vi "BUILD_install and upload core.vi"(7 "buildlog":path, 9 "LabVIEW Version":string, 10 "Repository Name":string, 11 "appended path":path) -> (0 "error out":errorcluster)   [LabVIEW 2013]
uses:
  <vilib>/JKI/VIPM API/VIPM API_vipm_api.lvlib
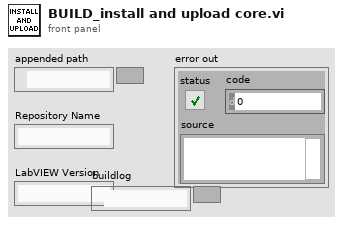
[diagram p1: front panel]
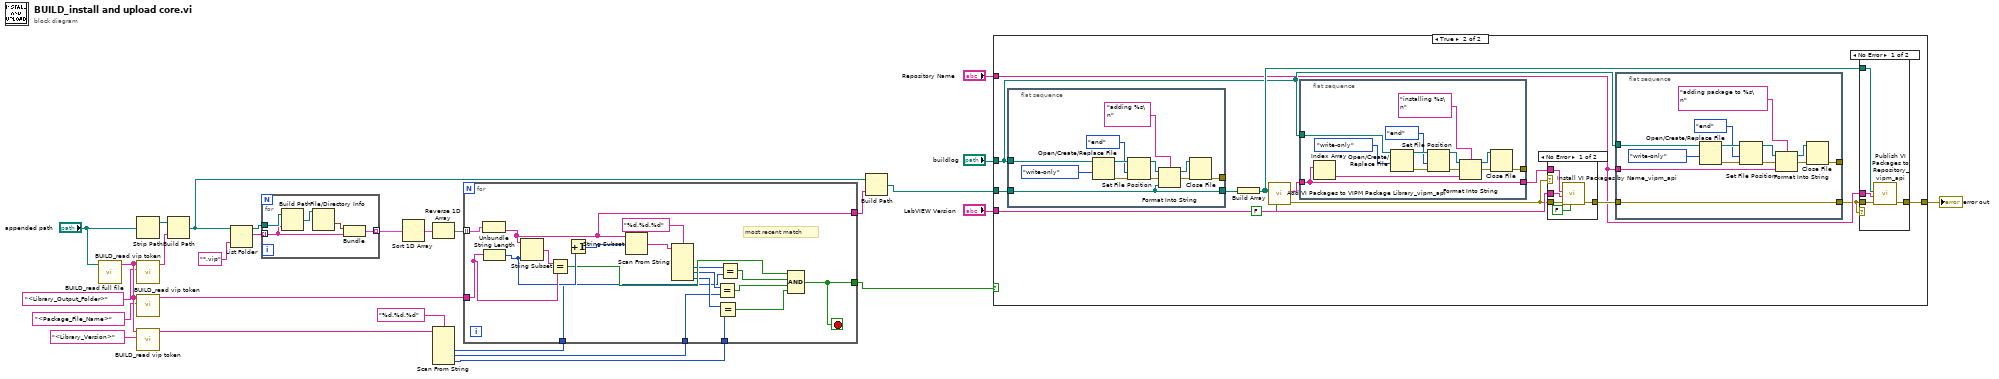
[diagram p0: block diagram]
diagram:
  n1 = call "BUILD_read full file.vi"("vip file"="appended path") -> ("data"=w23:string)  [unwired: 9 in, 1 out]
  n2 = Strip Path(path="appended path") -> (stripped path=w27:path)  [unwired: 1 out]
  n3 = call "BUILD_read vip token.vi"("regular expression"="<Library_Output_Folder>", "data"=w23) -> ("trimmed string"=w17:string)  [unwired: 9 in]
  n4 = call "BUILD_read vip token.vi"("regular expression"="<Package_File_Name>", "data"=w23) -> ("trimmed string"=w21:string)  [unwired: 9 in]
  n5 = call "BUILD_read vip token.vi"("regular expression"="<Library_Version>", "data"=w23) -> ("trimmed string"=w19:string)  [unwired: 9 in]
  n6 = Build Path(base path=w27, name or relative path=w17) -> (appended path=w13:path)
  n7 = List Folder(path=w13, pattern="*.vip") -> (path out=w3:path, filenames=w4:string[])  [unwired: 2 in, 2 out]
  n8 = for {
    tunnel: w3 -> [w32]
    tunnel: w4 -> [w29] mode=indexing
    tunnel: [w28] -> w5 mode=indexing
    n9 = Build Path(base path=w32, name or relative path=w29) -> (appended path=w31:path)
    n10 = File/Directory Info(path=w31) -> (last mod=w30:timestamp)  [unwired: 1 in, 6 out]
    n11 = Bundle("last mod"=w30, w29) -> (w28:cluster{"last mod":timestamp, string})  [unwired: 1 in]
  }
  n12 = Sort 1D Array(array=w5) -> (sorted array=w6:cluster{"last mod":timestamp, string}[])
  n13 = Reverse 1D Array(array=w6) -> (reversed array=w7:cluster{"last mod":timestamp, string}[])
  n14 = Scan From String(format string="%d.%d.%d", input string=w19) -> (output 1=w9:i32, output 2=w10:i32, output 3=w11:i32)  [unwired: 5 in, 3 out]
  n15 = for {
    tunnel: w7 -> [w51] mode=indexing
    tunnel: w21 -> [w49]
    tunnel: w9 -> [w37]
    tunnel: w10 -> [w36]
    tunnel: w11 -> [w35]
    tunnel: [w34] -> w12
    tunnel: [w33] -> w14
    stop <- w33 stop-if-true
    # "most recent match"
    n16 = Unbundle(w51) -> (w34:string)  [unwired: 1 out]
    n17 = String Length(string=w49) -> (length=w47:i32)
    n18 = String Subset(string=w34, length (rest)=w47) -> (substring=w50:string)  [unwired: 1 in]
    n19 = Equal?(x=w50, y=w49) -> (x = y?=w44:bool)
    n20 = Increment(x=w47) -> (x+1=w48:i32)
    n21 = String Subset(string=w34, offset (0)=w48) -> (substring=w46:string)  [unwired: 1 in]
    n22 = Scan From String(format string="%d.%d.%d", input string=w46) -> (output 1=w40:i32, output 2=w39:i32, output 3=w38:i32)  [unwired: 5 in, 3 out]
    n23 = Equal?(x=w39, y=w36) -> (x = y?=w42:bool)
    n24 = Equal?(x=w38, y=w35) -> (x = y?=w41:bool)
    n25 = Equal?(x=w40, y=w37) -> (x = y?=w43:bool)
    n26 = Compound Arithmetic op=AND(w44, w43, w42, w41) -> (w33:bool)
  }
  n27 = Build Path(base path=w13, name or relative path=w12) -> (appended path=w15:path)
  n28 = case shown="True" w14 {
    tunnel: w15 -> [_ w61]
    tunnel: [_ w63] -> w16
    tunnel: "LabVIEW Version" -> [_ w62]
    tunnel: "Repository Name" -> [_ w55]
    tunnel: "buildlog" -> [_ w59]
    frame False {
    }
    frame True {
      n29 = flat-sequence {
        tunnel: [w105] -> _
        tunnel: w61 -> [w104]
        tunnel: [w104] -> w60
        tunnel: w59 -> [w102]
        frame #0 {
          n30 = Open/Create/Replace File(file path (use dialog)=w102, access (0:read/write)=enum16{"read/write", "read-only", "write-only"}."write-only") -> (refnum out=w113:refnum<file>, error out=w112:errorcluster)  [unwired: 4 in, 1 out]
          n31 = Set File Position(refnum=w113, from (0:start)=enum16{"start", "end", "current"}."end", error in=w112) -> (refnum out=w111:refnum<file>, error out=w110:errorcluster)  [unwired: 1 in]
          n32 = Format Into String(format string="adding %s\n", initial string=w111, error in=w110, w104) -> (resulting string=w109:refnum<file>, error out=w108:errorcluster)
          n33 = Close File(refnum=w109, error in=w108) -> (error out=w105:errorcluster)  [unwired: 1 out]
        }
      }
      n34 = Build Array(w60) -> (w64:path[])
      n35 = call <vilib>:"Add VI Packages to VIPM Package Library_vipm_api.vi"("quiet? (T)"=FALSE, "Packages to add to VIPM Library (vipc,vip,ogp)"=w64) -> ("error out"=w54:errorcluster, "Package Names Added"=w58:string[])  [unwired: 8 in]
      n36 = flat-sequence {
        tunnel: [w93] -> _
        tunnel: w59 -> [w91]
        tunnel: w58 -> [w89]
        tunnel: [w89] -> w57
        frame #0 {
          n37 = Index Array(array=w89) -> (element=w90:string)  [unwired: 1 in]
          n38 = Open/Create/Replace File(file path (use dialog)=w91, access (0:read/write)=enum16{"read/write", "read-only", "write-only"}."write-only") -> (refnum out=w101:refnum<file>, error out=w100:errorcluster)  [unwired: 4 in, 1 out]
          n39 = Set File Position(refnum=w101, from (0:start)=enum16{"start", "end", "current"}."end", error in=w100) -> (refnum out=w99:refnum<file>, error out=w98:errorcluster)  [unwired: 1 in]
          n40 = Format Into String(format string="installing %s\n", initial string=w99, error in=w98, w90) -> (resulting string=w97:refnum<file>, error out=w96:errorcluster)
          n41 = Close File(refnum=w97, error in=w96) -> (error out=w93:errorcluster)  [unwired: 1 out]
        }
      }
      n42 = case shown="No Error" w54 {
        tunnel: w62 -> [w74 _]
        tunnel: w57 -> [w73 _]
        tunnel: [w72 w75] -> w56
        tunnel: w54 -> [w71 w75]
        frame No Error {
          n43 = call <vilib>:"Install VI Packages by Name_vipm_api.vi"("quiet? (T)"=FALSE, "error in (no error)"=w71, "LabVIEW Version"=w74, "Package Names to Install []"=w73) -> ("error out"=w72:errorcluster)  [unwired: 7 in]
        }
        frame Error {
        }
      }
      n44 = flat-sequence {
        tunnel: [w80] -> _
        tunnel: w59 -> [w78]
        tunnel: [w77] -> w53
        tunnel: w56 -> [w77]
        tunnel: w55 -> [w76]
        frame #0 {
          n45 = Open/Create/Replace File(file path (use dialog)=w78, access (0:read/write)=enum16{"read/write", "read-only", "write-only"}."write-only") -> (refnum out=w88:refnum<file>, error out=w87:errorcluster)  [unwired: 4 in, 1 out]
          n46 = Set File Position(refnum=w88, from (0:start)=enum16{"start", "end", "current"}."end", error in=w87) -> (refnum out=w86:refnum<file>, error out=w85:errorcluster)  [unwired: 1 in]
          n47 = Format Into String(format string="adding package to %s\n", initial string=w86, error in=w85, w76) -> (resulting string=w84:refnum<file>, error out=w83:errorcluster)
          n48 = Close File(refnum=w84, error in=w83) -> (error out=w80:errorcluster)  [unwired: 1 out]
        }
      }
      n49 = case shown="No Error" w53 {
        tunnel: w64 -> [w68 _]
        tunnel: [w67 w69] -> w63
        tunnel: w53 -> [w66 w69]
        tunnel: w55 -> [w65 _]
        frame No Error {
          n50 = call <vilib>:"Publish VI Packages to Repository_vipm_api.vi"("error in (no error)"=w66, "Repository Name"=w65, "Packages to publish to Repository Library (vip,ogp)"=w68) -> ("error out"=w67:errorcluster)  [unwired: 7 in, 1 out]
        }
        frame Error {
        }
      }
    }
  }
  "error out" <- w16
